vi "NumIntegrate_Trap_Dbl.vi"(8 "dT":dbl=0.02, 9 "Prev Y":dbl, 10 "Y":dbl, 11 "Prev Integral":dbl) -> (1 "New Prev Y":dbl, 3 "Integral":dbl)   [LabVIEW 2019, in "Trajectory_Library.lvlib"]
doc: "Performs the calculation for trapezoidal integration. The previous value of X is not stored inside this function The user is responsible for this.\n\nInputs:\n - Prev_Integral -- The previous value of the integrated value\n - Y -- Current value of Y\n - Prev Y -- The previous value of Y.\n - dT -- Time interval over which to integrate\n\nOutputs:\n - Integral -- Updated integrated output\n - New Prev Y -- The previous value of Y to use the next iteration."
uses:
  Trajectory_Library.lvlib
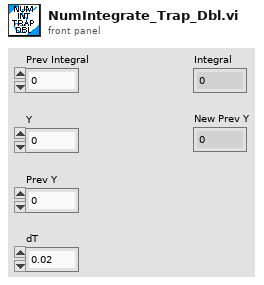
[diagram p1: front panel]
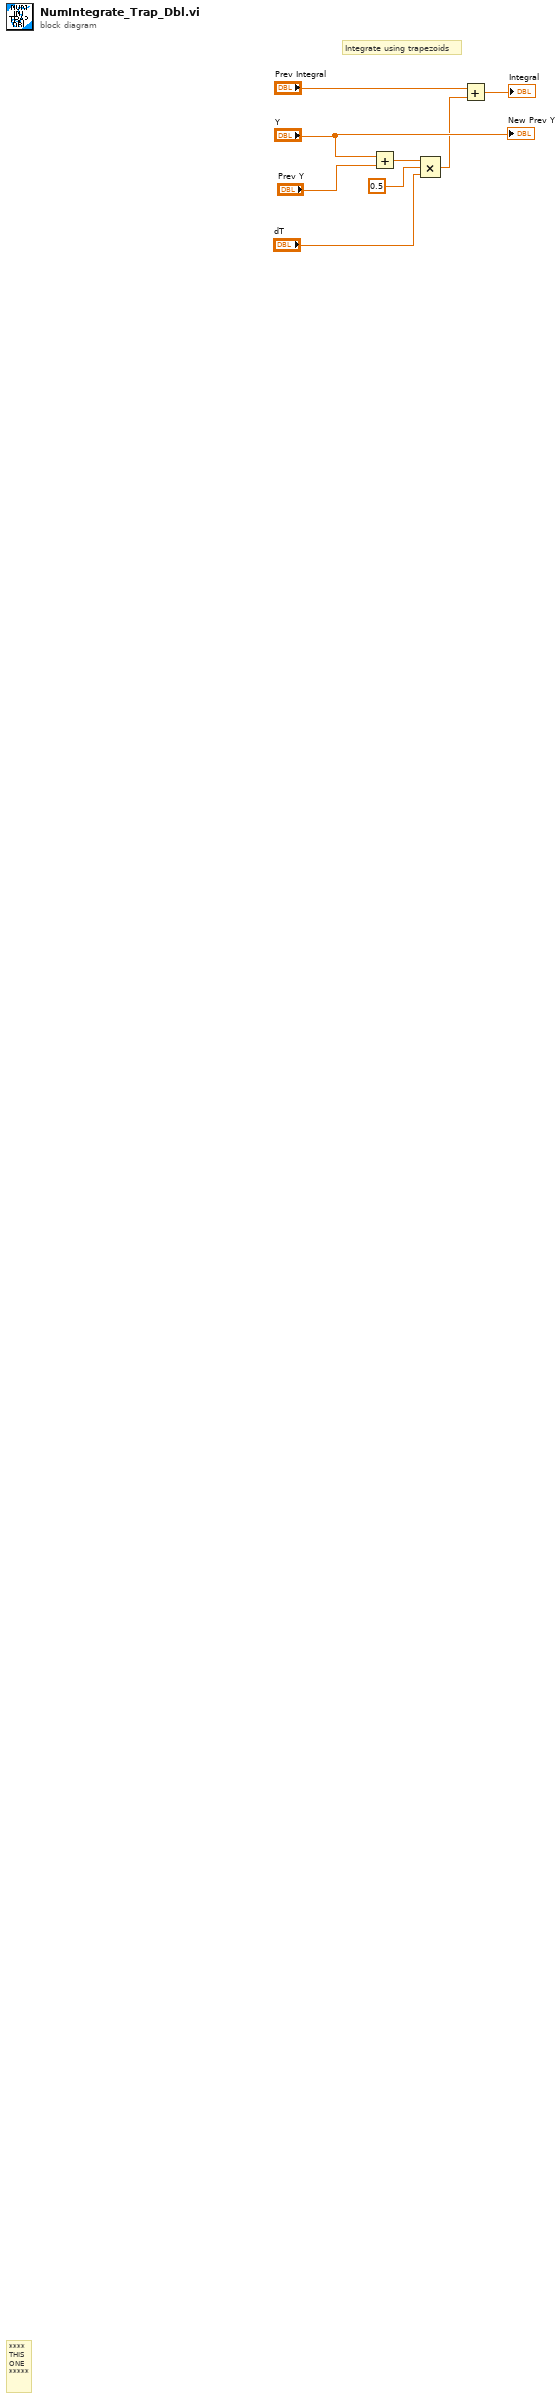
[diagram p0: block diagram]
diagram:
  # "Integrate using trapezoids"
  # "****\nTHIS\nONE\n*****"
  n1 = Add(x="Y", y="Prev Y") -> (x+y=w7:dbl)
  n2 = Compound Arithmetic op=MULTIPLY(w7, 0.5 ("value"), "dT") -> (w3:dbl)
  n3 = Add(x="Prev Integral", y=w3) -> (x+y=→"Integral":dbl)
  "New Prev Y" <- "Y"
